vi "Fetch Waveforms.vi"(8 "error in (no error)":errorcluster, 11 "OWON SDS1022 in":refnum<class "OWON SDS1022.lvclass">) -> (0 "error out":errorcluster, 3 "OWON SDS1022 out":refnum<class "OWON SDS1022.lvclass">)   [LabVIEW 2023, in "OWON SDS1022.lvlib" / "OWON SDS1022.lvclass"]
uses:
  OWON SDS1022.lvclass
  OWON SDS1022.lvclass/OWON SDS1022.ctl
  HAL/Scope Base/Scope Base.lvclass
  HAL/Interfaces/IConfigure Scope/IConfigure Scope.lvclass
  E:/git/HAL/Scope VISA/Scope VISA.lvclass
  E:/git/HAL/Scope Base/Scope Base.lvclass
  E:/git/HAL/Hardware_class/Instrument.lvclass
  E:/git/HAL/Interfaces/IScope/IScope.lvclass
  E:/git/OWON-SDS1022-LabVIEW/OWON SDS1022/OWON SDS1022.lvclass
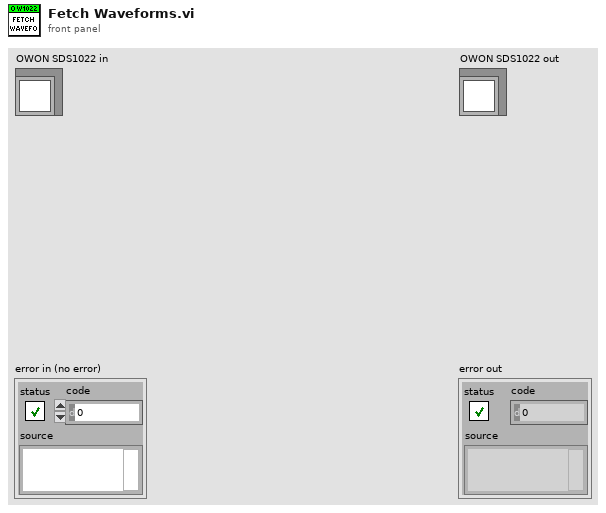
[diagram p1: front panel]
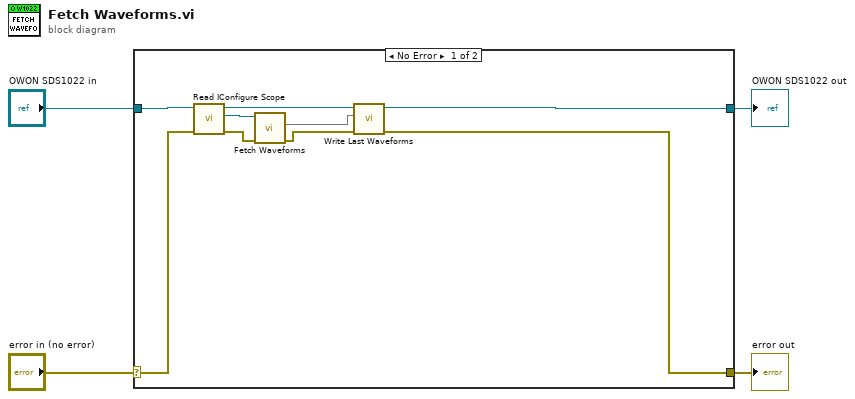
[diagram p0: block diagram]
diagram:
  n1 = case shown="No Error" "error in (no error)" {
    selector: "error in (no error)" -> [w13 w15]
    tunnel: [w8 w15] -> w3
    tunnel: [w6 w14] -> w1
    tunnel: "OWON SDS1022 in" -> [w12 w14]
    frame No Error {
      n2 = call "Read IConfigure Scope.vi"("error in (no error)"=w13, "Scope Base in"=w12) -> ("error out"=w10:errorcluster, "IConfigureScope"=w11:refnum<class "IConfigure Scope.lvclass">, "Scope Base out"=w7:refnum<class "OWON SDS1022.lvclass">)  [unwired: 7 in]
      n3 = call-dynamic "Fetch Waveforms.vi"("error in (no error)"=w10, "IConfigure Scope in"=w11) -> ("error out"=w9:errorcluster, "Last Waveforms"=w5:map{u8, waveform(dbl)})  [unwired: 7 in, 1 out]
      n4 = call "Write Last Waveforms.vi"("error in (no error)"=w9, "Last Waveforms"=w5, "Scope Base in"=w7) -> ("error out"=w8:errorcluster, "Scope Base out"=w6:refnum<class "OWON SDS1022.lvclass">)  [unwired: 7 in]
    }
    frame Error {
    }
  }
  "error out" <- w3
  "OWON SDS1022 out" <- w1
